vi "TimeResponse.vi"(8 "error in (no error)":errorcluster, 10 "SignalIn.lvclass in":refnum<class "SignalIn.lvclass">, 11 "System.lvclass in":refnum<class "System.lvclass">) -> (0 "error out":errorcluster, 1 "Simulation Graph":cluster{"time":dbl[], dbl[]}[](graph), 2 "SignalIn.lvclass out":refnum<class "SignalIn.lvclass">, 3 "System.lvclass out":refnum<class "System.lvclass">, 4 "Simulation Data":T1={"Time"=[], "Outputs Data"=[], "States Data"=[], "plot type"=enum."simulation"} {"States Data" format="%#.6g"; "Outputs Data" format="%#.6g"; "Time" format="%#.6g"})   [LabVIEW 2011, in "System.lvclass"]
uses:
  System.lvclass
  <vilib>/addons/Control Design/_Model Construction/NI_LinSys_Model Creation.lvlib
  <vilib>/addons/Control Design/_Model Construction/Model Creation.llb/Model Creation SubVI/cd_Create Transfer Function Model.vi
  <vilib>/addons/Control Design/_Time Response Analysis/NI_CD_Time Response.lvlib
  <vilib>/addons/Control Design/_Time Response Analysis/Time Response.llb/Time Response subVI/cd_Linear Simulation (Transfer Function).vi
  <vilib>/addons/Control Design/_Model Construction/Data Typedefs.llb/CD Plot Types Enum.ctl
  <vilib>/addons/Control Design/_Model Construction/NI_LinSys_Data Typedefs.lvlib
  <vilib>/addons/Control Design/_Model Construction/Data Typedefs.llb/CD MIMO Time Response Data.ctl
  SignalIn/SignalIn.lvclass
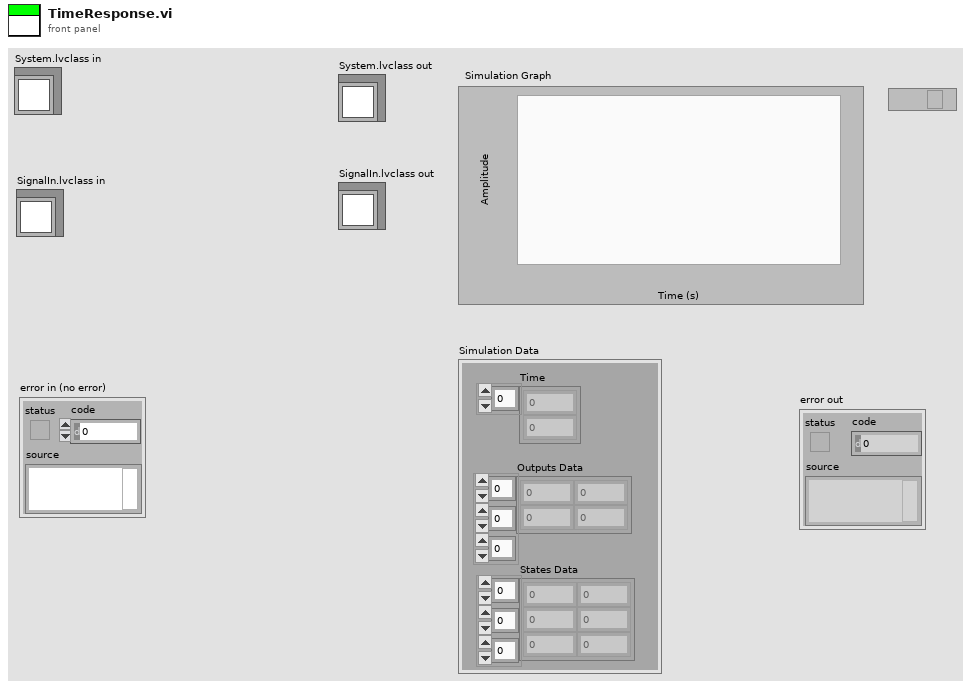
[diagram p1: front panel]
types:
  T1 = typedef "NI_LinSys_Data Typedefs.lvlib/CD MIMO Time Response Data.ctl" = cluster{"Time":dbl[], "Outputs Data":dbl[][][], "States Data":dbl[][][], "plot type":T2}
  T2 = typedef "NI_LinSys_Data Typedefs.lvlib/CD Plot Types Enum.ctl" = enum16{"bode-magnitude", "bode-phase", "nichols", "nyquist", "singular values", "step", "impulse", "initial", "simulation"}
  T3 = typedef "NI_LinSys_Model Typedefs.lvlib/CD Transfer Function Model (MIMO).ctl" = cluster{"properties":T4, "transfer function(s)":T5[][]}
  T4 = typedef "NI_LinSys_Model Typedefs.lvlib/CD General Elements.ctl" = cluster{"Model name":string, "Input names":string[], "Output names":string[], "Input Delays":dbl[], "Output Delays":dbl[], "Sampling Time":dbl, "Notes":string}
  T5 = typedef "NI_LinSys_Model Typedefs.lvlib/CD Transfer Function Model (SISO).ctl" = cluster{"Numerator":dbl[], "Denominator":dbl[], "delay":dbl}
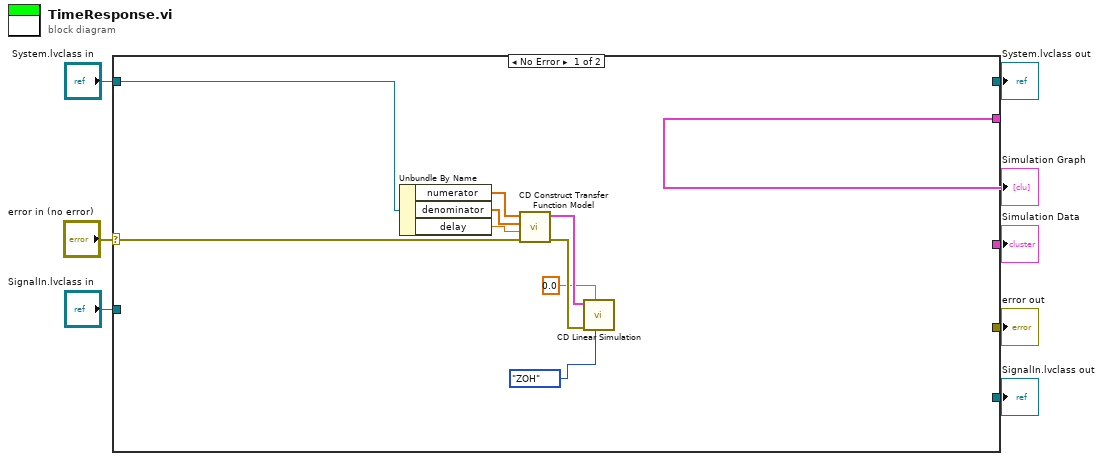
[diagram p0: block diagram]
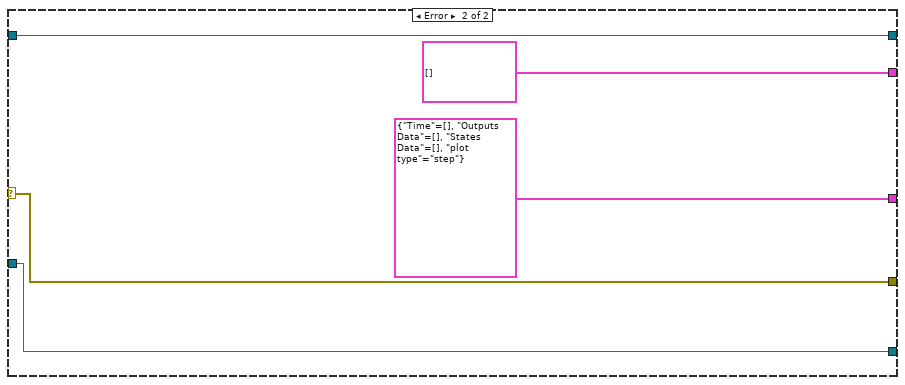
[diagram p2: hidden frame]
diagram:
  n1 = case shown="No Error" "error in (no error)" {
    selector: "error in (no error)" -> [w11 w20]
    tunnel: "SignalIn.lvclass in" -> [_ w21]
    tunnel: [_ w21] -> w7
    tunnel: [_ w20] -> w6
    tunnel: [_ cluster{"time":dbl[], dbl[]}[] [] ("Simulation Graph")] -> w5
    tunnel: [_ T1 {"Time"=[], "Outputs Data"=[], "States Data"=[], "plot type"=enum."step"} ("Simulation Data")] -> w4
    tunnel: [_ w22] -> w2
    tunnel: "System.lvclass in" -> [w10 w22]
    frame No Error {
      n2 = Unbundle By Name(w10) -> ("numerator"=w17:dbl[], "denominator"=w16:dbl[], "delay"=w15:dbl)
      n3 = call-poly <vilib>:"CD Construct Transfer Function Model.vi"("error in (no error)"=w11, "Delay"=w15, "Denominator"=w16, "Numerator"=w17) -> ("error out"=w13:errorcluster, "Transfer Function Model"=w14:T3)  [unwired: 6 in]
      n4 = call-poly <vilib>:"CD Linear Simulation.vi"("Method"=enum16{"ZOH", "FOH"}."ZOH", "Initial time"=0.0, "error in (no error)"=w13, "Transfer Function Model"=w14) -> ()  [unwired: 5 in, 3 out]
    }
    frame Error {
    }
  }
  "System.lvclass out" <- w2
  "SignalIn.lvclass out" <- w7
  "error out" <- w6
  "Simulation Graph" <- w5
  "Simulation Data" <- w4
